vi "SetExposure.vi"(8 "error in":errorcluster, 10 "Exp":u32, 11 "camera.nit in":refnum<class "camera.lvclass">) -> (0 "error out":errorcluster)   [LabVIEW 2020, in "camera.lvclass"]
uses:
  camera.lvclass
  f8a5b868-a8bf-4099-a5bd-ecbad76ba6b9.vi
  camera.lvclass/camera.ctl
  lib/O-PL.dll
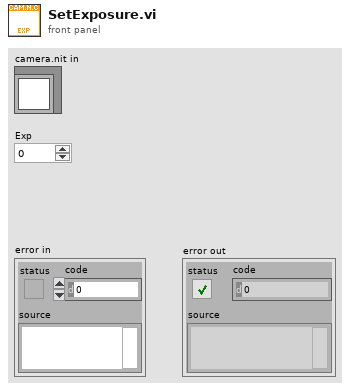
[diagram p1: front panel]
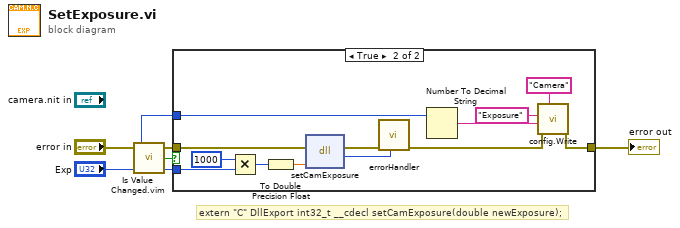
[diagram p0: block diagram]
diagram:
  # "extern \"C\" DllExport int32_t __cdecl setCamExposure(double newExposure);"
  n1 = call "Is Value Changed.vim"("value"="Exp") -> ("changed or first call?"=w4:bool)
  n2 = case shown="True" w4 {
    tunnel: "Exp" -> [_ w17]
    tunnel: "error in" -> [w5 w16]
    tunnel: [w5 w8] -> w2
    tunnel: "Exp" -> [_ w6]
    frame False {
    }
    frame True {
      n3 = Multiply(x=u32 1000 ("y"), y=w17) -> (x*y=w15:u32)
      n4 = To Double Precision Float(number=w15) -> (double precision float=w14:dbl)
      n5 = dll-call lib="C:/Users/pittsburger.SOLARIS/Desktop/v0.8/lib/O-PL.dll" fn="setCamExposure"(error in=w16, "exposure"=w14) -> (error out=w13:errorcluster, "return type"=w12:i32)  [unwired: 3 in, 1 out]
      n6 = call "errorHandler.vi"("code"=w12, "error in"=w13) -> ("error out"=w9:errorcluster)  [unwired: 9 in]
      n7 = Number To Decimal String(number=w6) -> (decimal integer string=w7:string)  [unwired: 1 in]
      n8 = call "config.Write.vi"("section"="Camera", "error in"=w9, "value"=w7, "key"="Exposure") -> ("error out"=w8:errorcluster)  [unwired: 7 in]
    }
  }
  "error out" <- w2
